vi "StoreDisplayImageReference.vi"(0 "object in":refnum<class "Hamamatsu.lvclass">, 2 "Image Src":T1, 5 "error in (no error)":errorcluster) -> (14 "object out":refnum<class "Hamamatsu.lvclass">, 16 "Image Dst Out":T1, 19 "error out":errorcluster)   [LabVIEW 2021, in "Hamamatsu.lvclass"]
uses:
  Hamamatsu.lvclass
  <vilib>/vision/Image Controls.llb/IMAQ Image.ctl
  Hamamatsu.lvclass/Hamamatsu.ctl
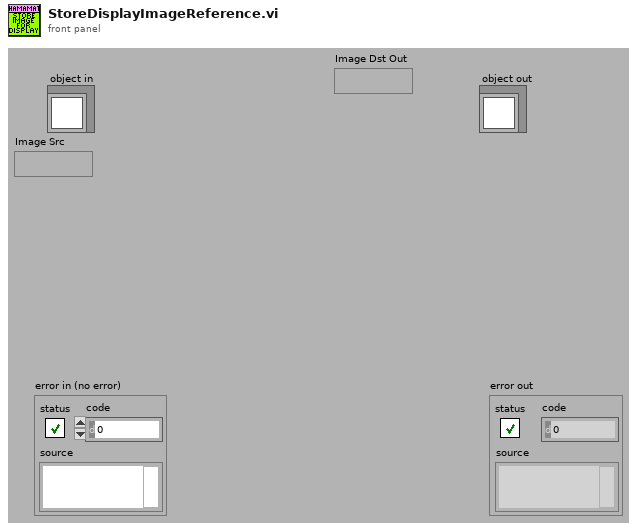
[diagram p1: front panel]
types:
  T1 = typedef "IMAQ Image.ctl" = refnum<image>
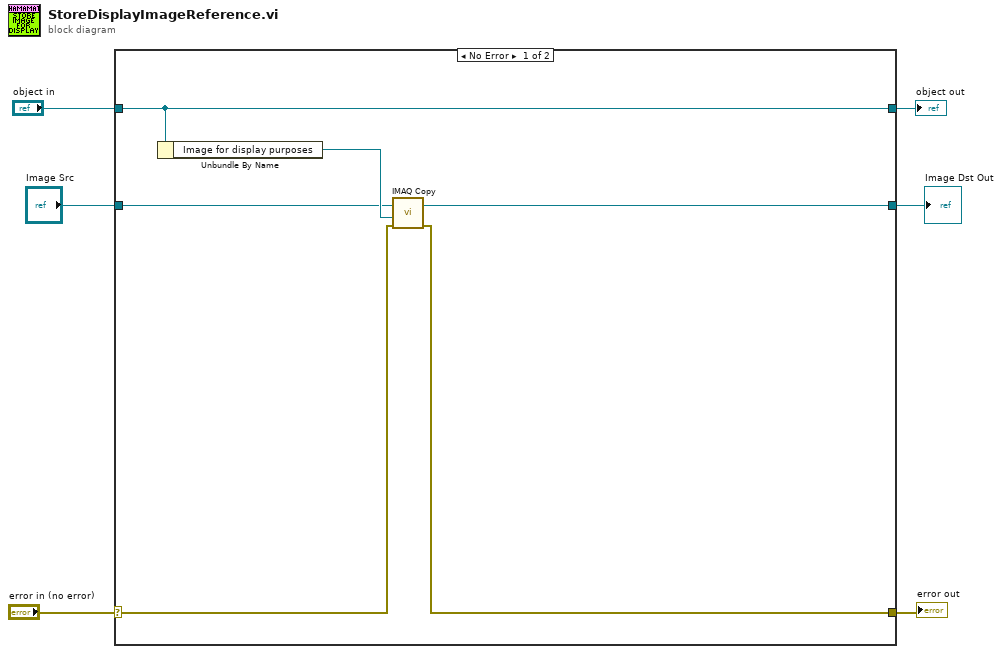
[diagram p0: block diagram]
diagram:
  n1 = case shown="No Error" "error in (no error)" {
    selector: "error in (no error)" -> [w8 w14]
    tunnel: [w7 w14] -> w5
    tunnel: [w12 w13] -> w3
    tunnel: "object in" -> [w12 w13]
    tunnel: [w10 _] -> w2
    tunnel: "Image Src" -> [w9 _]
    frame No Error {
      n2 = Unbundle By Name(w12) -> ("Image for display purposes"=w11:T1)
      n3 = call "IMAQ Copy"("error in (no error)"=w8, "Image Dst"=w11, "Image Src"=w9) -> ("error out"=w7:errorcluster, "Image Dst Out"=w10:T1)  [unwired: 3 in]
    }
    frame Error {
    }
  }
  "error out" <- w5
  "object out" <- w3
  "Image Dst Out" <- w2
